vi "Stack Tote2.vi"(8 "error in (no error)":errorcluster, 9 "Auto Notifiers In":T2, 11 "End at":T1=enum."Tote 2") -> (0 "error out":errorcluster, 1 "Auto Notifiers Out":T2)   [LabVIEW 2014]
doc: "This VI will set the elevator to the input state and then set the arm rollers to spin outward to prepare for contact with recycling bin"
uses:
  Auto Notifiers.ctl
  Main/Arms/Arm clapper state.ctl
  Main/Arms/Arm State.ctl
  Main/Elevator/Elevator States.ctl
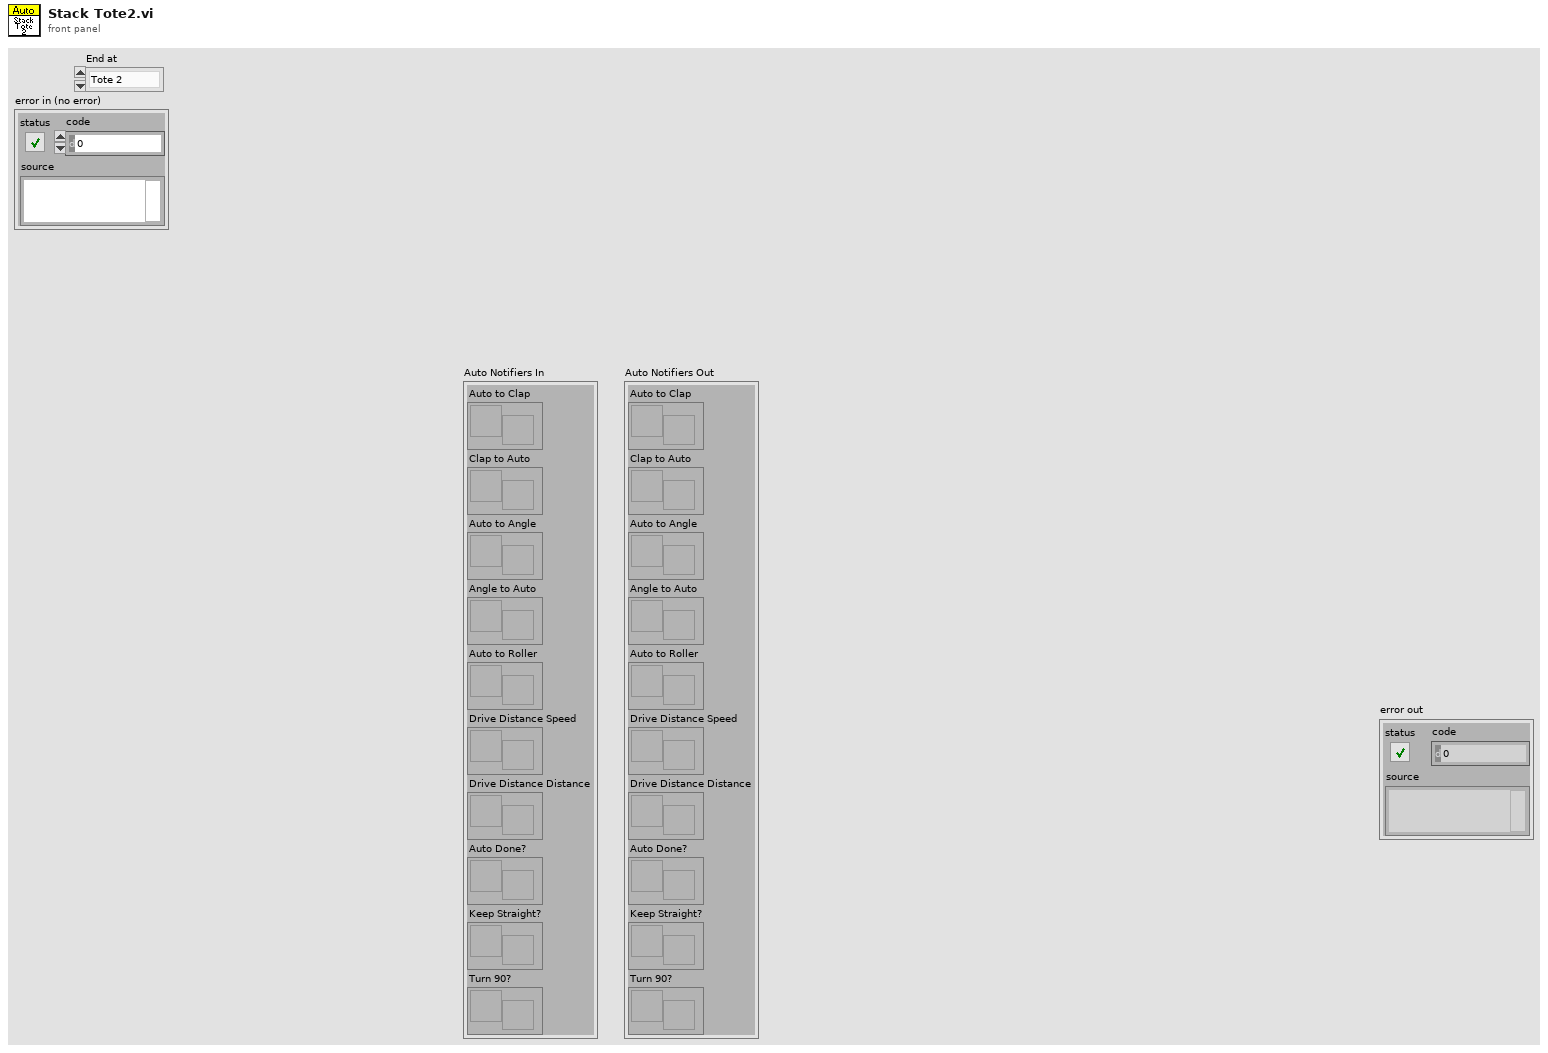
[diagram p1: front panel]
types:
  T1 = typedef "Elevator States.ctl" = enum16{"Ground", "Tote 1", "Tote 2", "Tote 3", "Tote 4", "Tote 5", "Tote 6"}
  T2 = typedef "Auto Notifiers.ctl" = cluster{"Auto to Clap":refnum<notifier>, "Clap to Auto":refnum<notifier>, "Auto to Angle":refnum<notifier>, "Angle to Auto":refnum<notifier>, "Auto to Roller":refnum<notifier>, "Drive Distance Speed":refnum<notifier>, "Drive Distance Distance":refnum<notifier>, "Auto Done?":refnum<notifier>, "Keep Straight?":refnum<notifier>, "Turn 90?":refnum<notifier>}
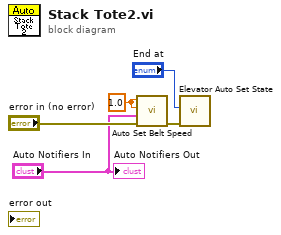
[diagram p0: block diagram]
diagram:
  w4 = 1.0 ("Right Belt")
  n1 = call "Auto Set Belt Speed.vi"("error in"="error in (no error)", "Auto Notifiers In"="Auto Notifiers In", "Right Belt"=w4, "Left Belt"=w4) -> ("error out"=w2:errorcluster)  [unwired: 6 in, 1 out]
  n2 = call "Elevator Auto Set State.vi"("error in (no error)"=w2, "New State"="End at") -> ()  [unwired: 9 in, 1 out]
  "Auto Notifiers Out" <- "Auto Notifiers In"
